vi "ConfigureDevice.vi"(11 "ContextIn":T8={"COMHandler"="", "HelloResponse"="", "FTDIDetected"=FALSE, "DeviceDetected"=FALSE, "TransferRefusedByUser"=FALSE, "AvailablePacketsNr"=0, "RequestType"=enum."NONE", "Response"="", "Packet(s)Available"=FALSE, "DownloadSuccess"=FALSE, "AppendDonwloadedPackets"=FALSE, "AppendLoadedPackets"=FALSE, "CfgDevWhenAvailable"=FALSE, "Packets"=[], "COMConfig"={"BaudRate"=9600, "DataBits"=8, "Parity"=enum."None", "StopBits"=10, "DataTransferTimeout[ms]"=10000, "FastTransferTimeout[ms]"=100, "ConnTries"=0, "MsWaitBeforeRetry"=0}, "ActivePacketID"=0, "AccelData"=[], "GyroData"=[], "ActiveMeasurementConfig"={"Frequency"=100, "Resolution[b]"=16, "AccelFSRange"=enum."+/-8g", "GyroFSRange"=enum."+/-1000dps"}, "OkayResponse"="", "MenuTags"={"SavePacketsTag"="", "ExportToCSVTag"="", "ExportToJSONTag"="", "ConfigureDeviceTag"="", "OpenPacketsTag"="", "OpenAndAppendPacketsTag"="", "EditCommentTag"="", "TakeGraphsScreenshotTag"=""}} {"ActiveMeasurementConfig"."Resolution[b]" min=4 max=16 step=1; "ActiveMeasurementConfig"."Frequency" min=1 max=10000000 step=1; "Packets"."MeasurementConfig"."Resolution[b]" min=4 max=16 step=1; "Packets"."MeasurementConfig"."Frequency" min=1 max=10000000 step=1; "COMConfig"."StopBits" items=["1.0"=10, "1.5"=15, "2.0"=20]; "COMConfig"."DataBits" min=7 max=9 step=1; "COMConfig"."BaudRate" min=9600 max=921600 step=1}) -> (3 "ContextOut":T8={"COMHandler"="", "HelloResponse"="", "FTDIDetected"=FALSE, "DeviceDetected"=FALSE, "TransferRefusedByUser"=FALSE, "AvailablePacketsNr"=0, "RequestType"=enum."NONE", "Response"="", "Packet(s)Available"=FALSE, "DownloadSuccess"=FALSE, "AppendDonwloadedPackets"=FALSE, "AppendLoadedPackets"=FALSE, "CfgDevWhenAvailable"=FALSE, "Packets"=[], "COMConfig"={"BaudRate"=9600, "DataBits"=8, "Parity"=enum."None", "StopBits"=10, "DataTransferTimeout[ms]"=10000, "FastTransferTimeout[ms]"=100, "ConnTries"=0, "MsWaitBeforeRetry"=0}, "ActivePacketID"=0, "AccelData"=[], "GyroData"=[], "ActiveMeasurementConfig"={"Frequency"=100, "Resolution[b]"=16, "AccelFSRange"=enum."+/-8g", "GyroFSRange"=enum."+/-1000dps"}, "OkayResponse"="", "MenuTags"={"SavePacketsTag"="", "ExportToCSVTag"="", "ExportToJSONTag"="", "ConfigureDeviceTag"="", "OpenPacketsTag"="", "OpenAndAppendPacketsTag"="", "EditCommentTag"="", "TakeGraphsScreenshotTag"=""}} {"ActiveMeasurementConfig"."Resolution[b]" min=4 max=16 step=1; "ActiveMeasurementConfig"."Frequency" min=1 max=10000000 step=1; "Packets"."MeasurementConfig"."Resolution[b]" min=4 max=16 step=1; "Packets"."MeasurementConfig"."Frequency" min=1 max=10000000 step=1; "COMConfig"."StopBits" items=["1.0"=10, "1.5"=15, "2.0"=20]; "COMConfig"."DataBits" min=7 max=9 step=1; "COMConfig"."BaudRate" min=9600 max=921600 step=1})   [LabVIEW 2016]
uses:
  FSContext.ctl
  Requests/RequestType.ctl
  Packet.ctl
  Sample.ctl
  Reading.ctl
  MeasurementConfig.ctl
  Measurement/AccelFSRange.ctl
  Measurement/GyroFSRange.ctl
  FTDI/COMConfig.ctl
  MenuTags.ctl
  ConfigureDevice/CDAccelFSRange.ctl
  ConfigureDevice/CDGyroFSRange.ctl
  ConfigureDevice/CDOutputDataRate.ctl
  ConfigureDevice/CDAccelDLPF.ctl
  ConfigureDevice/CDGyroDLPF.ctl
  ConfigureDevice/CDInterruptPinMode.ctl
  ConfigureDevice/CDInterruptMode.ctl
  ConfigureDevice/CDState.ctl
  ConfigureDevice/CDSensorConfiguration.ctl
  ConfigureDevice/CDContext.ctl
  JSON/JSONStreamType.ctl
  <vilib>/event_ctls.llb/eventvkey.ctl
  <vilib>/addons/JSON API/JSON Value/Set from JSON string.vi
  <vilib>/addons/JSON API/JSON Value/JSON Value.lvclass
  <vilib>/addons/JSON API/Get Polymorphic/JSON GetSet.lvlib
panel:
  out "Resolution [b]":u32=4 min=16 max=16 step=1
  in  "Interrupt Mode":T1
  in  "Interrupt Pin Mode":T2
  in  "GyroDLPF":T3
  in  "AccelDLPF":T4
  in  "Output Data Rate":T5
  in  "GyroFSRange":T6
  in  "AccelFSRange":T7
  in  "ConfigureButton":bool
  in  "CloseButton":bool
  # "Acquistion"
  # "Accelerometer"
  # "Gyroscope"
  # "Full Scale Range"
  # "Digital Lowpass Filter Frequency"
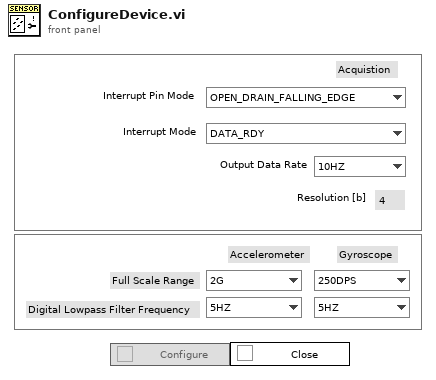
[diagram p1: front panel]
types:
  T1 = typedef "CDInterruptMode.ctl" = enum16{"DATA_RDY"}
  T2 = typedef "CDInterruptPinMode.ctl" = enum16{"OPEN_DRAIN_FALLING_EDGE"}
  T3 = typedef "CDGyroDLPF.ctl" = enum16{"5HZ", "10HZ", "20HZ", "41HZ", "92HZ", "184HZ"}
  T4 = typedef "CDAccelDLPF.ctl" = enum16{"5HZ", "10HZ", "20HZ", "41HZ", "92HZ", "184HZ", "460HZ"}
  T5 = typedef "CDOutputDataRate.ctl" = enum16{"10HZ", "20HZ", "40HZ", "50HZ", "100HZ", "200HZ", "500HZ", "1000HZ"}
  T6 = typedef "CDGyroFSRange.ctl" = enum16{"250DPS", "500DPS", "1000DPS", "2000DPS"}
  T7 = typedef "CDAccelFSRange.ctl" = enum16{"2G", "4G", "8G", "16G"}
  T8 = typedef "FSContext.ctl" = cluster{"COMHandler":refnum<visa-resource-name>, "HelloResponse":string, "FTDIDetected":bool, "DeviceDetected":bool, "TransferRefusedByUser":bool, "AvailablePacketsNr":u32, "RequestType":T9, "Response":string, "Packet(s)Available":bool, "DownloadSuccess":bool, "AppendDonwloadedPackets":bool, "AppendLoadedPackets":bool, "CfgDevWhenAvailable":bool, "Packets":T10[], "COMConfig":T16, "ActivePacketID":i32, "AccelData":waveform(dbl)[], "GyroData":waveform(dbl)[], "ActiveMeasurementConfig":T13, "OkayResponse":string, "MenuTags":T17}
  T9 = typedef "RequestType.ctl" = enum16{"NONE", "Reset", "Hello", "GetPacketsNr", "GetPacket", "GetConfig", "SetConfig", "SendConfig", "Goodbye"}
  T10 = typedef "Packet.ctl" = cluster{"ID":u32, "SamplesNr":u32, "Samples":T11[], "MeasurementConfig":T13, "Comment":string}
  T11 = typedef "Sample.ctl" = cluster{"Accel":T12, "Gyro":T12}
  T12 = typedef "Reading.ctl" = cluster{"X":i16, "Y":i16, "Z":i16}
  T13 = typedef "MeasurementConfig.ctl" = cluster{"Frequency":u32, "Resolution[b]":u32, "AccelFSRange":T14, "GyroFSRange":T15}
  T14 = typedef "AccelFSRange.ctl" = enum16{"+/-2g", "+/-4g", "+/-8g", "+/-16g"}
  T15 = typedef "GyroFSRange.ctl" = enum16{"+/-250dps", "+/-500dps", "+/-1000dps", "+/-2000dps"}
  T16 = typedef "COMConfig.ctl" = cluster{"BaudRate":u32, "DataBits":u16, "Parity":enum16{"None", "Odd", "Even", "Mark", "Space"}, "StopBits":u16, "DataTransferTimeout[ms]":u32, "FastTransferTimeout[ms]":u32, "ConnTries":i32, "MsWaitBeforeRetry":u32}
  T17 = typedef "MenuTags.ctl" = cluster{"SavePacketsTag":string, "ExportToCSVTag":string, "ExportToJSONTag":string, "ConfigureDeviceTag":string, "OpenPacketsTag":string, "OpenAndAppendPacketsTag":string, "EditCommentTag":string, "TakeGraphsScreenshotTag":string}
  T18 = typedef "CDContext.ctl" = cluster{"CfgRcvSuccessfully":bool, "CfgSending":bool, "CfgSentSuccessfully":bool}
  T19 = typedef "CDSensorConfiguration.ctl" = cluster{"AccelFSRange":T7, "GyroFSRange":T6, "ODR":T5, "AccelDLPF":T4, "GyroDLPF":T3, "InterruptPinMode":T2, "InterruptMode":T1, "Resolution":u32}
  T20 = typedef "CDState.ctl" = enum16{"IDLE", "HandleErrors", "WaitForEvent", "Init", "GetSensorConfig", "InformAboutCfgRxSuccess", "ConfigureSensor", "InformAboutCfgTxSuccess", "UpdateUI", "Stop"}
  T21 = enum8{"Enabled", "Disabled", "Disabled and Grayed Out"}
  T22 = typedef "JSONStreamType.ctl" = enum16{"Raw", "Pretty"}
  T23 = typedef "eventvkey.ctl" = enum16{"ASCII", "Enter", "Return", "Shift", "Ctrl", "Alt", "Cmd", "Opt", "Caps", "NumLock", "Clear", "Break", "Up", "Down", "Left", "Right", "Insert", "Delete", "Home", "End", "PageUp", "PageDown", "Escape", "Help", "Pause", "ScrollLock", "F1", "F2", "F3", "F4", "F5", "F6", "F7", "F8", "F9", "F10", "F11", "F12", "F13", "F14", "F15", "F16", "F17", "F18", "F19", "F20", "F21", "F22", "F23", "F24", "Play", "VolumeUp", "VolumeDown", "Mute", "Two Byte Char"}
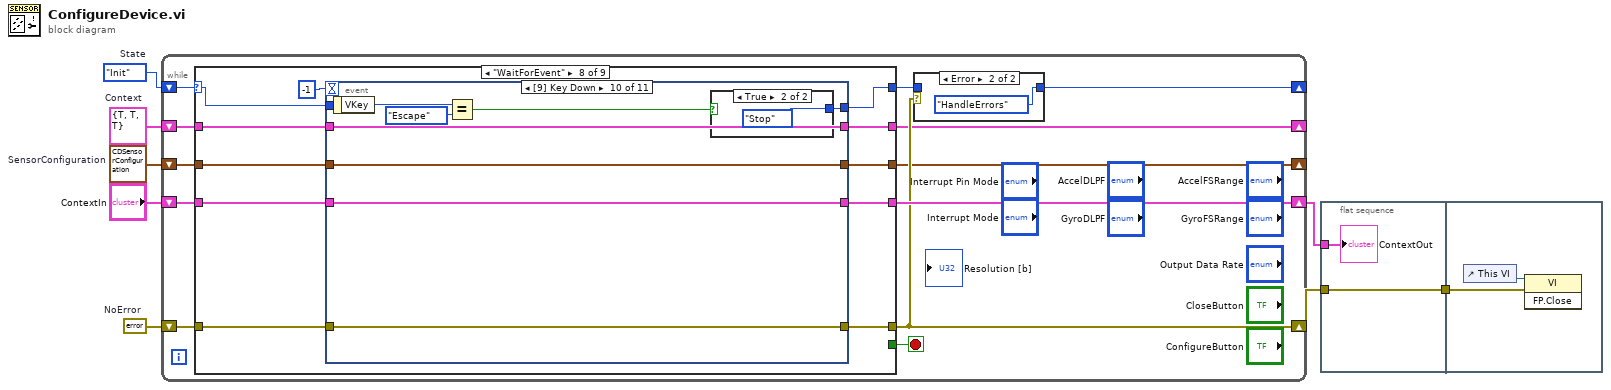
[diagram p0: block diagram]
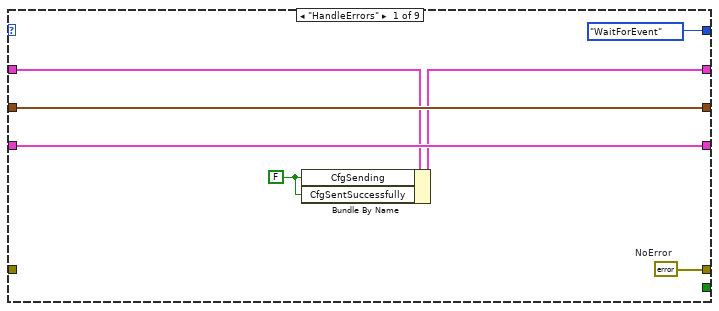
[diagram p3: hidden frame]
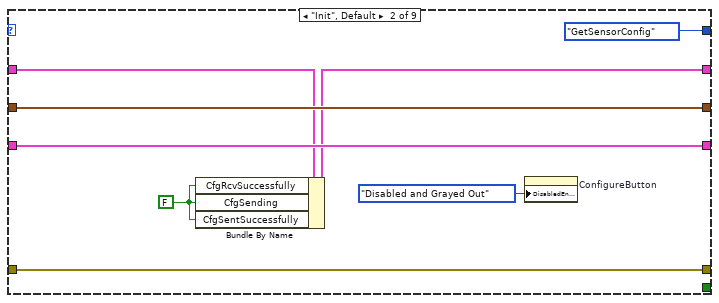
[diagram p4: hidden frame]
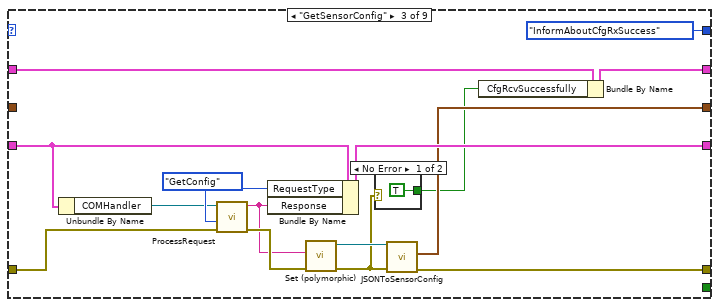
[diagram p5: hidden frame]
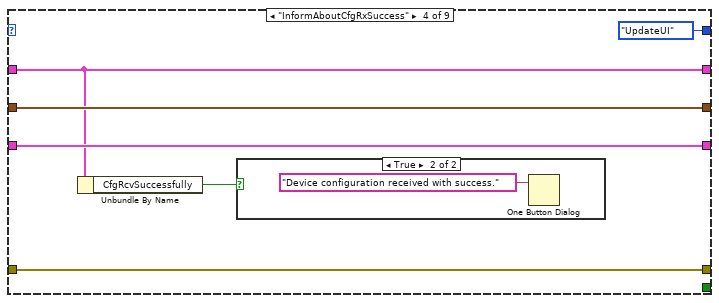
[diagram p7: hidden frame]
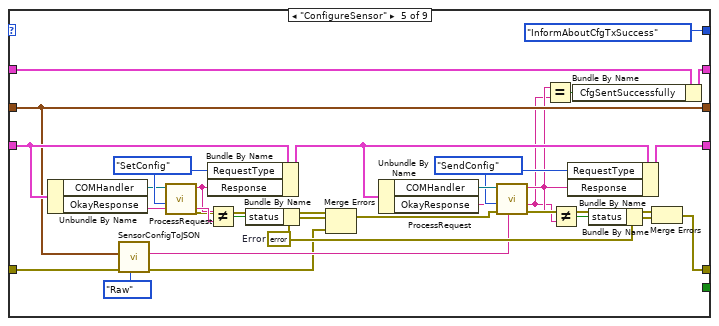
[diagram p9: hidden frame]
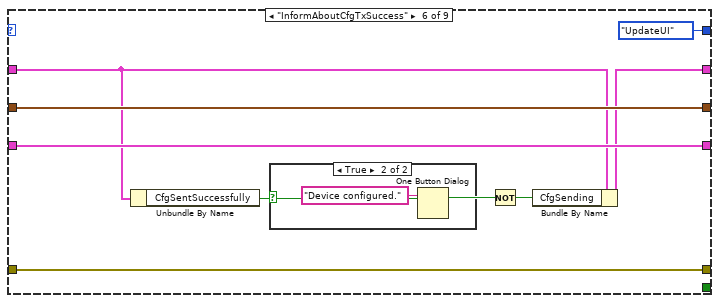
[diagram p10: hidden frame]
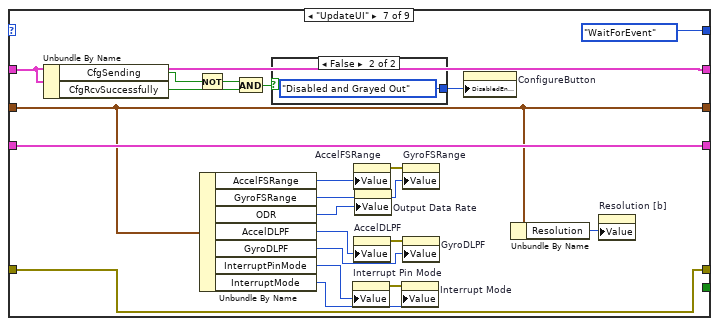
[diagram p12: hidden frame]
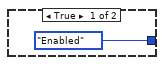
[diagram p13: hidden frame]
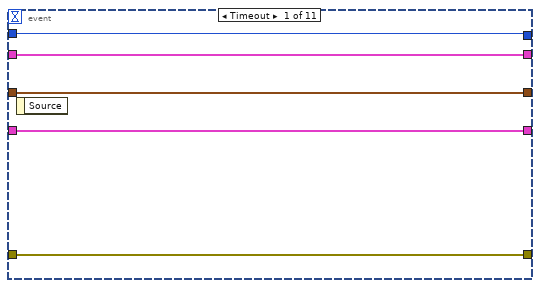
[diagram p14: hidden frame]
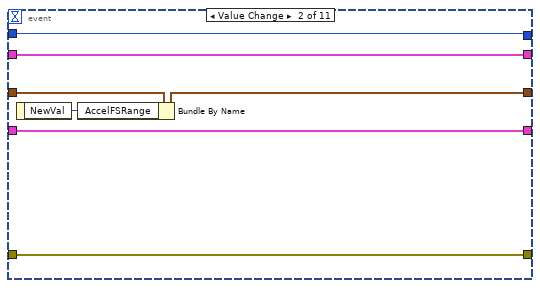
[diagram p15: hidden frame]
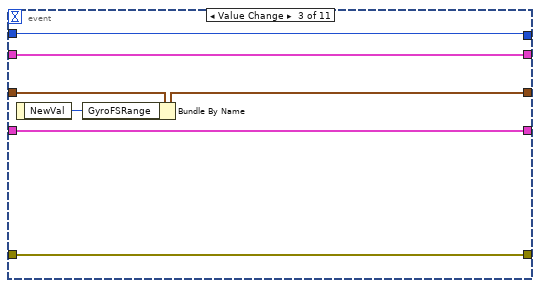
[diagram p16: hidden frame]
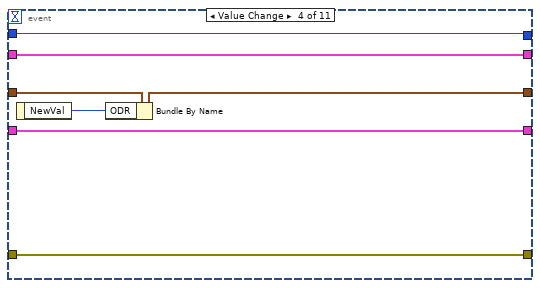
[diagram p17: hidden frame]
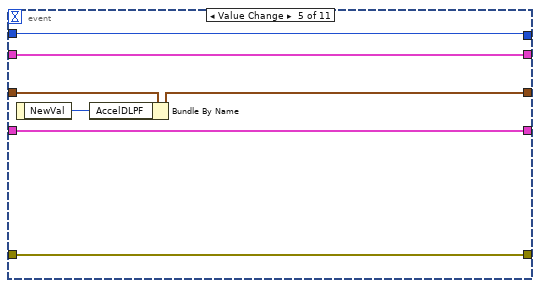
[diagram p18: hidden frame]
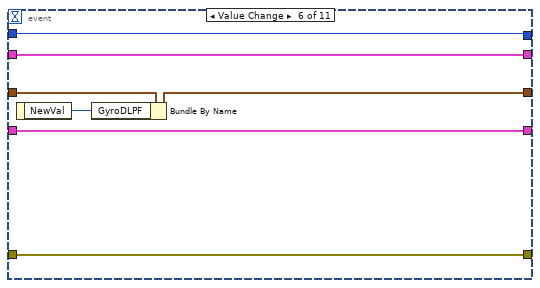
[diagram p19: hidden frame]
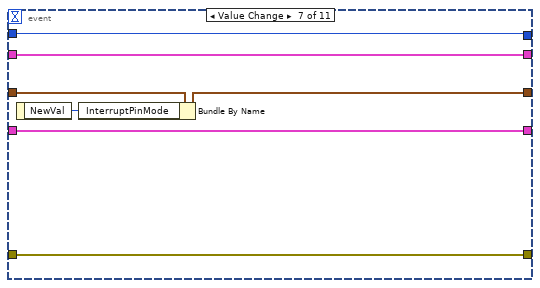
[diagram p20: hidden frame]
diagram:
  w1 = T18 {"CfgRcvSuccessfully"=TRUE, "CfgSending"=TRUE, "CfgSentSuccessfully"=TRUE}  # Context
  w3 = T19 {"AccelFSRange"=enum."2G", "GyroFSRange"=enum."250DPS", "ODR"=enum."10HZ", "AccelDLPF"=enum."5HZ", "GyroDLPF"=enum."5HZ", "InterruptPinMode"=enum."OPEN_DRAIN_FALLING_EDGE", "InterruptMode"=enum."DATA_RDY", "Resolution"=4}  # SensorConfiguration
  w6 = errorcluster {"status"=FALSE, "code"=0, "source"=""}  # NoError
  w7 = CDState."Init"  # State
  n1 = while {
    shift-right: [w18] -> w2
    shift-left: "ContextIn" -> [w19]
    shift-right: [w16] -> _
    shift-left: w7 -> [w20]
    shift-right: [w12] -> w4
    shift-left: w6 -> [w17]
    shift-right: [w11] -> _
    shift-left: w3 -> [w15]
    shift-right: [w9] -> _
    shift-left: w1 -> [w10]
    stop <- w13 stop-if-true
    n2 = case shown="\"WaitForEvent\"" w20 {
      selector: w20 -> [_ _ _ _ _ _ _ w129 w212]
      tunnel: w19 -> [w29 w36 w48 w58 w82 w96 w118 w126 w211]
      tunnel: [w29 w36 w49 w58 w73 w96 w118 w125 w211] -> w18
      tunnel: w17 -> [_ w37 w50 w59 w89 w97 w107 w128 w213]
      tunnel: [w27 w37 w44 w59 w70 w97 w107 w127 w213] -> w12
      tunnel: w15 -> [w28 w34 _ w57 w66 w95 w99 w131 w210]
      tunnel: [CDState."WaitForEvent" ("State") CDState."GetSensorConfig" ("State") CDState."InformAboutCfgRxSuccess" ("State") CDState."UpdateUI" ("State") CDState."InformAboutCfgTxSuccess" ("State") CDState."UpdateUI" ("State") CDState."WaitForEvent" ("State") w130 w212] -> w14
      tunnel: [_ _ _ _ _ _ _ _ TRUE] -> w13
      tunnel: [w28 w34 w43 w57 w66 w95 w99 w124 w210] -> w11
      tunnel: w10 -> [w25 w32 w42 w55 w65 w92 w106 w123 w209]
      tunnel: [w24 w31 w41 w55 w64 w91 w106 w122 w209] -> w9
      frame "HandleErrors" {
        w23 = FALSE ("CfgSending")
        w27 = errorcluster {"status"=FALSE, "code"=0, "source"=""}  # NoError
        n3 = Bundle By Name(cluster=w25, "CfgSending"=w23, "CfgSentSuccessfully"=w23) -> (w24:T18)
      }
      frame "Init", Default {
        w30 = FALSE ("CfgSending")
        n4 = Bundle By Name(cluster=w32, "CfgRcvSuccessfully"=w30, "CfgSending"=w30, "CfgSentSuccessfully"=w30) -> (w31:T18)
        n5 = property on="ConfigureButton" class="Bool"("DisabledEnum"=T21."Disabled and Grayed Out" ("Disabled")) -> ()  [unwired: 2 in, 2 out]
      }
      frame "GetSensorConfig" {
        w52 = RequestType."GetConfig" ("RequestType")
        n6 = Unbundle By Name(w48) -> ("COMHandler"=w51:refnum<visa-resource-name>)
        n7 = call "ProcessRequest.vi"("ErrorIn"=w50, "RequestType"=w52, "DeviceResourceName"=w51) -> ("ErrorOut"=w47:errorcluster, "Response"=w46:string)  [unwired: 5 in, 2 out]
        n8 = Bundle By Name(cluster=w48, "RequestType"=w52, "Response"=w46) -> (w49:T8)
        n9 = call-poly <vilib>:"Set (polymorphic).vi"("error in (no error)"=w47, "JSON stream"=w46) -> ("error out"=w39:errorcluster, "JSON Value out"=w45:refnum<class "JSON Value.lvclass">)  [unwired: 7 in, 1 out]
        n10 = case shown="No Error" w39 {
          tunnel: [TRUE _] -> w38
          frame No Error {
          }
          frame Error {
          }
        }
        n11 = call "JSONToSensorConfig.vi"("ErrorIn"=w39, "JSONIn"=w45) -> ("ErrorOut"=w44:errorcluster, "SensorConfiguration"=w43:T19)  [unwired: 7 in, 1 out]
        n12 = Bundle By Name(cluster=w42, "CfgRcvSuccessfully"=w38) -> (w41:T18)
      }
      frame "InformAboutCfgRxSuccess" {
        n13 = Unbundle By Name(w55) -> ("CfgRcvSuccessfully"=w54:bool)
        n14 = case shown="True" w54 {
          frame False {
          }
          frame True {
            n15 = One Button Dialog(message="Device configuration received with success.") -> ()  [unwired: 1 in, 1 out]
          }
        }
      }
      frame "ConfigureSensor" {
        w81 = RequestType."SendConfig" ("RequestType")
        w79 = errorcluster {"status"=FALSE, "code"=0, "source"="Invalid okay response"}  # Error
        w88 = RequestType."SetConfig" ("RequestType")
        n16 = Unbundle By Name(w82) -> ("COMHandler"=w87:refnum<visa-resource-name>, "OkayResponse"=w86:string)
        n17 = call "SensorConfigToJSON.vi"("StreamType"=JSONStreamType."Raw", "ErrorIn"=w89, "SensorConfig"=w66) -> ("ErrorOut"=w68:errorcluster, "JSONSensorConfig"=w69:string)  [unwired: 6 in, 1 out]
        n18 = call "ProcessRequest.vi"("RequestType"=w88, "DeviceResourceName"=w87) -> ("ErrorOut"=w77:errorcluster, "Response"=w85:string)  [unwired: 6 in, 2 out]
        n19 = Bundle By Name(cluster=w82, "RequestType"=w88, "Response"=w85) -> (w72:T8)
        n20 = Not Equal?(x=w85, y=w86) -> (x != y?=w84:bool)
        n21 = Bundle By Name(cluster=w79, "status"=w84) -> (w76:errorcluster)
        n22 = Merge Errors(w77, w76, w68) -> (w78:errorcluster)
        n23 = Unbundle By Name(w72) -> ("COMHandler"=w83:refnum<visa-resource-name>, "OkayResponse"=w61:string)
        n24 = call "ProcessRequest.vi"("CustomMessage"=w69, "ErrorIn"=w78, "RequestType"=w81, "DeviceResourceName"=w83) -> ("ErrorOut"=w74:errorcluster, "Response"=w62:string)  [unwired: 4 in, 2 out]
        n25 = Equal?(x=w62, y=w61) -> (x = y?=w63:bool)
        n26 = Not Equal?(x=w62, y=w61) -> (x != y?=w80:bool)
        n27 = Bundle By Name(cluster=w72, "RequestType"=w81, "Response"=w62) -> (w73:T8)
        n28 = Bundle By Name(cluster=w65, "CfgSentSuccessfully"=w63) -> (w64:T18)
        n29 = Bundle By Name(cluster=w79, "status"=w80) -> (w75:errorcluster)
        n30 = Merge Errors(w74, w75) -> (w70:errorcluster)
      }
      frame "InformAboutCfgTxSuccess" {
        n31 = Unbundle By Name(w92) -> ("CfgSentSuccessfully"=w93:bool)
        n32 = case shown="True" w93 {
          frame False {
          }
          frame True {
            n33 = One Button Dialog(message="Device configured.") -> ()  [unwired: 1 in, 1 out]
          }
        }
        n34 = Not(x=w93) -> (.not. x?=w90:bool)
        n35 = Bundle By Name(cluster=w92, "CfgSending"=w90) -> (w91:T18)
      }
      frame "UpdateUI" {
        n36 = Unbundle By Name(w106) -> ("CfgSending"=w103:bool, "CfgRcvSuccessfully"=w102:bool)
        n37 = Not(x=w103) -> (.not. x?=w101:bool)
        n38 = Unbundle By Name(w99) -> ("AccelFSRange"=w117:T7, "GyroFSRange"=w116:T6, "ODR"=w114:T5, "AccelDLPF"=w112:T4, "GyroDLPF"=w111:T3, "InterruptPinMode"=w109:T2, "InterruptMode"=w108:T1)
        n39 = And(x=w101, y=w102) -> (x .and. y?=w104:bool)
        n40 = case shown="False" w104 {
          tunnel: [T21."Enabled" ("Disabled") T21."Disabled and Grayed Out" ("Disabled")] -> w105
          frame True {
          }
          frame False {
          }
        }
        n41 = property on="Interrupt Pin Mode" class="Enum (strict)"("Value"=w109) -> (error out=w110:errorcluster)  [unwired: 2 in, 1 out]
        n42 = property on="AccelFSRange" class="Enum (strict)"("Value"=w117) -> (error out=w115:errorcluster)  [unwired: 2 in, 1 out]
        n43 = property on="AccelDLPF" class="Enum (strict)"("Value"=w112) -> (error out=w113:errorcluster)  [unwired: 2 in, 1 out]
        n44 = property on="Output Data Rate" class="Enum (strict)"("Value"=w114) -> ()  [unwired: 2 in, 2 out]
        n45 = property on="Interrupt Mode" class="Enum (strict)"(error in=w110, "Value"=w108) -> ()  [unwired: 1 in, 2 out]
        n46 = property on="GyroFSRange" class="Enum (strict)"(error in=w115, "Value"=w116) -> ()  [unwired: 1 in, 2 out]
        n47 = property on="GyroDLPF" class="Enum (strict)"(error in=w113, "Value"=w111) -> ()  [unwired: 1 in, 2 out]
        n48 = property on="ConfigureButton" class="Bool"("DisabledEnum"=w105) -> ()  [unwired: 2 in, 2 out]
        n49 = Unbundle By Name(w99) -> ("Resolution"=w100:u32)
        n50 = property on="Resolution [b]" class="DigNum (strict)"("Value"=w100) -> ()  [unwired: 2 in, 2 out]
      }
      frame "WaitForEvent" {
        n51 = event shown="[9] Key Down" {
          selector: _ -> [_ _ _ _ _ _ _ _ _ _ _]
          dyn-events: _ -> [_ _ _ _ _ _ _ _ _ _ _]
          timeout: -1 -> [_ _ _ _ _ _ _ _ _ _ _]
          tunnel: w131 -> [w134 w143 w150 w157 w164 w171 w178 w185 w188 w196 w205]
          tunnel: [w137 w138 w145 w152 w159 w166 w173 w180 CDState."Stop" ("State") w199 CDState."ConfigureSensor" ("State")] -> w130
          tunnel: w129 -> [w137 w138 w145 w152 w159 w166 w173 w180 _ _ _]
          tunnel: w128 -> [w136 w140 w147 w154 w161 w168 w175 w182 w189 w197 w206]
          tunnel: [w136 w140 w147 w154 w161 w168 w175 w182 w189 w197 w206] -> w127
          tunnel: w126 -> [w135 w141 w148 w155 w162 w169 w176 w183 w190 w198 w207]
          tunnel: [w135 w141 w148 w155 w162 w169 w176 w183 w190 w198 w207] -> w125
          tunnel: [w134 w142 w149 w156 w163 w170 w177 w184 w188 w196 w205] -> w124
          tunnel: w123 -> [w133 w139 w146 w153 w160 w167 w174 w181 w187 w195 w204]
          tunnel: [w133 w139 w146 w153 w160 w167 w174 w181 w187 w195 w203] -> w122
          event Timeout {
            n52 = event-data() -> ()  [unwired: 1 in, 1 out]
          }
          event Value Change {
            n53 = event-data() -> ("NewVal"=w144:T7)  [unwired: 1 in]
            n54 = Bundle By Name(cluster=w143, "AccelFSRange"=w144) -> (w142:T19)
          }
          event Value Change {
            n55 = event-data() -> ("NewVal"=w151:T6)  [unwired: 1 in]
            n56 = Bundle By Name(cluster=w150, "GyroFSRange"=w151) -> (w149:T19)
          }
          event Value Change {
            n57 = event-data() -> ("NewVal"=w158:T5)  [unwired: 1 in]
            n58 = Bundle By Name(cluster=w157, "ODR"=w158) -> (w156:T19)
          }
          event Value Change {
            n59 = event-data() -> ("NewVal"=w165:T4)  [unwired: 1 in]
            n60 = Bundle By Name(cluster=w164, "AccelDLPF"=w165) -> (w163:T19)
          }
          event Value Change {
            n61 = event-data() -> ("NewVal"=w172:T3)  [unwired: 1 in]
            n62 = Bundle By Name(cluster=w171, "GyroDLPF"=w172) -> (w170:T19)
          }
          event Value Change {
            n63 = event-data() -> ("NewVal"=w179:T2)  [unwired: 1 in]
            n64 = Bundle By Name(cluster=w178, "InterruptPinMode"=w179) -> (w177:T19)
          }
          event Value Change {
            n65 = event-data() -> ("NewVal"=w186:T1)  [unwired: 1 in]
            n66 = Bundle By Name(cluster=w185, "InterruptMode"=w186) -> (w184:T19)
          }
          event "CloseButton": Value Change {
            n67 = event-data() -> ()  [unwired: 1 in, 1 out]
          }
          event Key Down {
            n68 = event-data() -> ("VKey"=w194:T23)  [unwired: 1 in]
            n69 = Equal?(x=w194, y=eventvkey."Escape") -> (x = y?=w192:bool)
            n70 = case shown="True" w192 {
              tunnel: [CDState."WaitForEvent" ("State") CDState."Stop" ("State")] -> w199
              frame False {
              }
              frame True {
              }
            }
          }
          event "ConfigureButton": Value Change {
            n71 = event-data() -> ()  [unwired: 1 in, 1 out]
            n72 = Bundle By Name(cluster=w204, "CfgSending"=TRUE) -> (w203:T18)
          }
        }
      }
      frame "Stop" {
      }
    }
    n73 = case shown="Error" w12 {
      tunnel: [w21 CDState."HandleErrors" ("State")] -> w16
      tunnel: w14 -> [w21 _]
      frame No Error {
      }
      frame Error {
      }
    }
  }
  n74 = flat-sequence {
    tunnel: w4 -> [w216]
    tunnel: [w216] -> w5
    tunnel: w2 -> [w215]
    tunnel: w5 -> [w217]
    frame #0 {
      "ContextOut" <- w215
    }
    frame #1 {
      n75 = control-ref of="This VI"() -> (w218:refnum<vi>)
      n76 = invoke class="VI" method="FP.Close"(reference=w218, error in=w217) -> ()  [unwired: 1 in, 3 out]
    }
  }
